vi "Arduino_v2.vi"() -> ()   [LabVIEW 2025]
uses:
  <vilib>/Instr/_visa.llb/VISA Configure Serial Port (Instr).vi
panel:
  out "Waveform Chart":dynamicdata(graph)
  out "datos":string
  in  "Kd":dbl(knob) scale=0.0..1.0
  in  "Ki":dbl(knob) scale=0.0..0.1
  in  "Kp":dbl(knob) scale=0.0..2.0
  out "posicion grafica":dbl(knob) scale=0.0..360.0
  out "Setpoint":dbl(knob) scale=0.0..360.0
  in  "OK Button":bool
  in  "Setpoint":string
  out "Posicion actual":i32
  out "Sensor":string
  in  "stop":bool
  in  "VISA resource name":refnum<visa-resource-name>
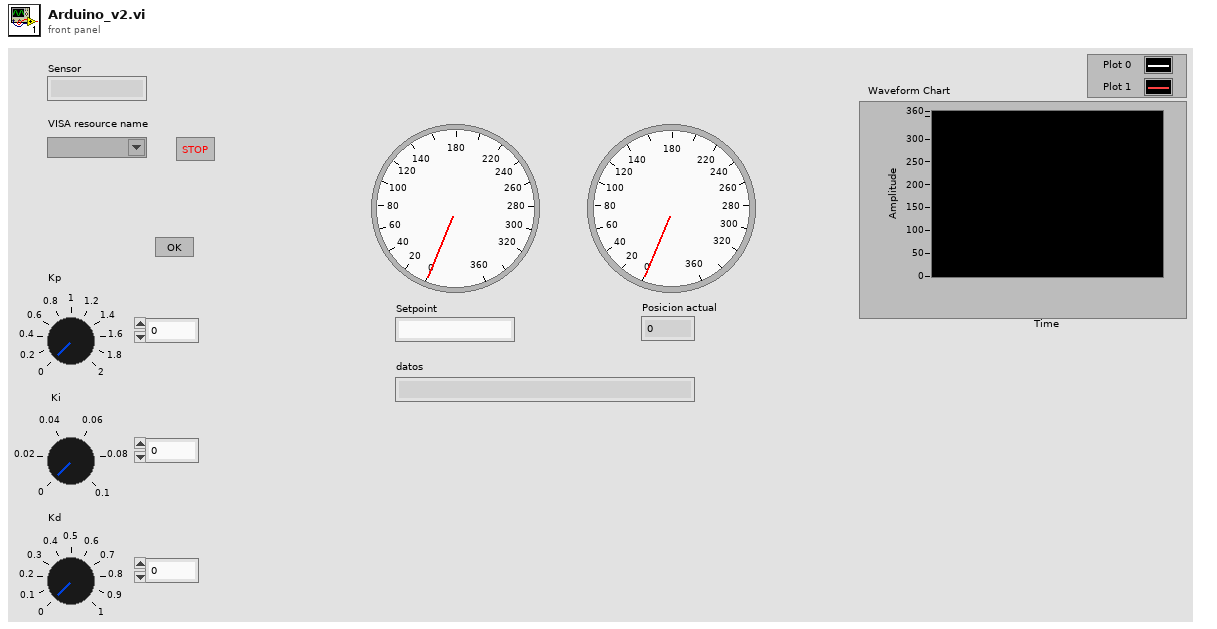
[diagram p1: front panel]
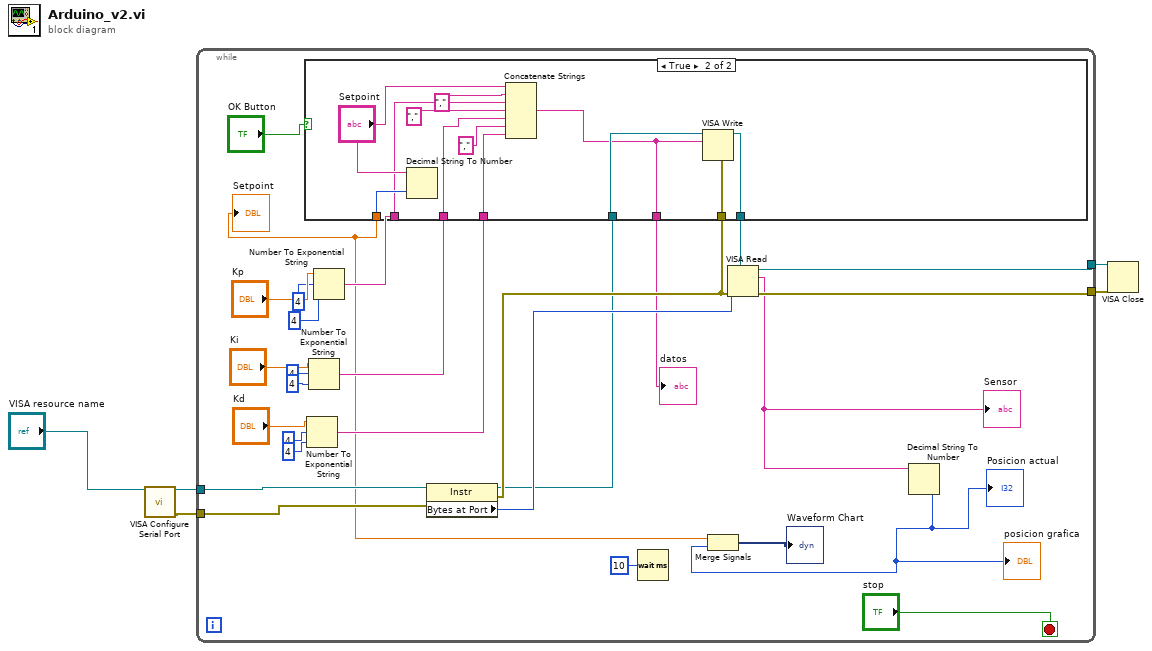
[diagram p0: block diagram]
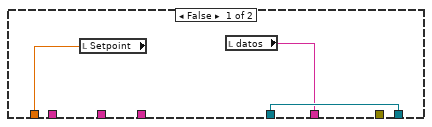
[diagram p2: hidden frame]
diagram:
  n1 = call-poly "VISA Configure Serial Port"("VISA resource name"="VISA resource name") -> ("VISA resource name out"=w4:refnum<visa-resource-name>, "error out"=w5:errorcluster)  [unwired: 13 in]
  n2 = while {
    tunnel: w5 -> [w32]
    tunnel: w4 -> [w26]
    tunnel: [w29] -> w3
    tunnel: [w30] -> w2
    stop <- "stop" stop-if-true
    n3 = Number To Exponential String(number="Kd", precision (6)=i16 4, 3:i16 4 ("precision (6)")) -> (E-format string=w16:string)  [unwired: 1 in]
    n4 = Number To Exponential String(number="Ki", precision (6)=i16 4, 3:i16 4 ("precision (6)")) -> (E-format string=w17:string)  [unwired: 1 in]
    n5 = Number To Exponential String(number="Kp", precision (6)=i16 4, 3:i16 4 ("precision (6)")) -> (E-format string=w18:string)  [unwired: 1 in]
    n6 = property class="Instr"(reference=w26, error in=w32) -> (reference out=w24:refnum<visa-resource-name>, error out=w25:errorcluster, "Bytes at Port"=w31:u32)
    n7 = case shown="True" "OK Button" {
      tunnel: w25 -> [_ w48]
      tunnel: w24 -> [w36 w47]
      tunnel: [w36 w46] -> w23
      tunnel: [w35 w45] -> w7
      tunnel: w18 -> [_ w42]
      tunnel: w17 -> [_ w40]
      tunnel: w16 -> [_ w38]
      tunnel: [w34 w37] -> w15
      frame False {
        n8 = local read "Setpoint"() -> (w35:dbl)
        n9 = local read "datos"() -> (w34:string)
      }
      frame True {
        n10 = Decimal String To Number(string="Setpoint") -> (number=w45:i32)  [unwired: 2 in, 1 out]
        n11 = Concatenate Strings("Setpoint", ",", w42, ",", w40, ",", w38) -> (w37:string)
        n12 = VISA Write(VISA resource name=w47, write buffer=w37, error in (no error)=w48) -> (VISA resource name out=w46:refnum<visa-resource-name>)  [unwired: 2 out]
      }
    }
    "Setpoint" <- w7
    "datos" <- w15
    n13 = Wait (ms)(milliseconds to wait=u32 10) -> ()  [unwired: 1 out]
    n14 = VISA Read(VISA resource name=w23, byte count=w31, error in (no error)=w25) -> (VISA resource name out=w29:refnum<visa-resource-name>, read buffer=w28:string, error out=w30:errorcluster)  [unwired: 1 out]
    "Sensor" <- w28
    n15 = Decimal String To Number(string=w28) -> (number=w6:i32)  [unwired: 2 in, 1 out]
    "Posicion actual" <- w6
    "posicion grafica" <- w6
    n16 = Merge Signals(w7, w6) -> (→"Waveform Chart":dynamicdata)
  }
  n17 = VISA Close(VISA resource name=w3, error in (no error)=w2) -> ()  [unwired: 1 out]
